vi "TRABS-calc.vi"(1 "I+II channel seq":T1) -> (0 "TRABS":dbl[](array[numeric]))   [LabVIEW 2015]
uses:
  controls/data-cluster.ctl
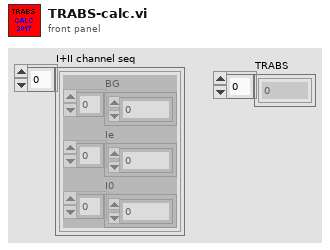
[diagram p1: front panel]
types:
  T1 = typedef "data-cluster.ctl" = cluster{"BG":i32[], "Ie":i32[], "I0":i32[]}[]
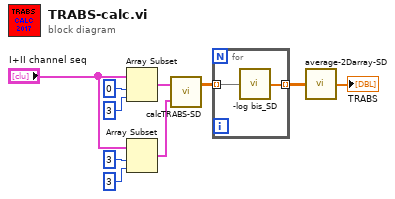
[diagram p0: block diagram]
diagram:
  n1 = Array Subset(array="I+II channel seq", index=0, length=3) -> (w2:T1)
  n2 = Array Subset(array="I+II channel seq", index=3, length=3) -> (w1:T1)
  n3 = call "calcTRABS-SD.vi"("II channel seq"=w1, "I channel seq"=w2) -> ("TRanS multiple measurements"=w9:dbl[][])  [unwired: 1 out]
  n4 = for {
    tunnel: w9 -> [w12] mode=indexing
    tunnel: [w11] -> w10 mode=indexing
    n5 = call "-log bis_SD.vi"("Transmission"=w12) -> ("-log(x)=log(1/x)"=w11:dbl[])
  }
  n6 = call "average-2Darray-SD.vi"("2D array"=w10) -> ("out array"=→"TRABS":dbl[])
